vi "Identify Duplicate Alias Entries.vi"(8 "error in (no error)":errorcluster, 10 "Modified Index":i32, 11 "NewVal":T1[](array[typedef])) -> (0 "error out":errorcluster, 1 "Duplicate Message":string, 2 "Duplicate Entry":bool)   [LabVIEW 2020, in "Routing and Faulting System Explorer.lvlib"]
uses:
  Routing and Faulting System Explorer.lvlib
  Alias.ctl
  Endpoint.ctl
  Shared/Constants.vi
  Shared/Routing and Faulting Shared.lvlib
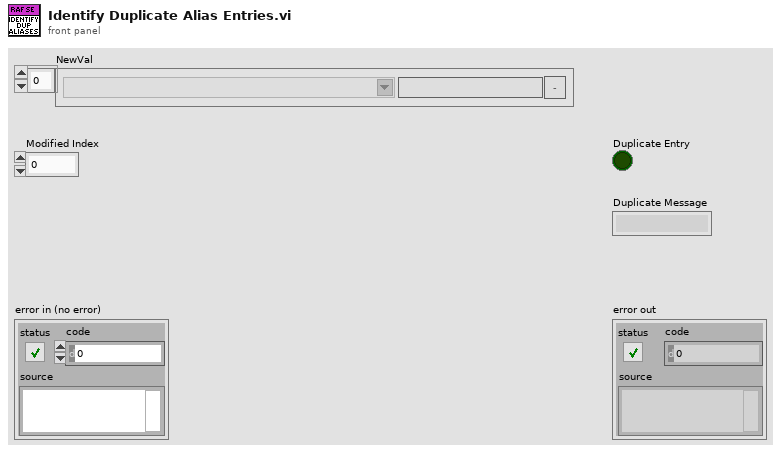
[diagram p1: front panel]
types:
  T1 = typedef "Routing and Faulting System Explorer.lvlib/Alias.ctl" = cluster{"Endpoint":T2, "Alias":string, "Remove":bool}
  T2 = typedef "Routing and Faulting System Explorer.lvlib/Endpoint.ctl" = string
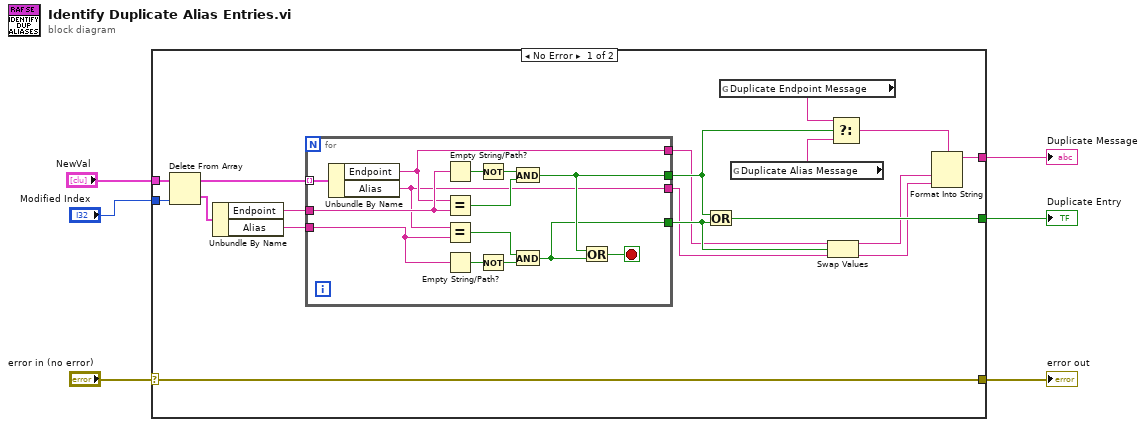
[diagram p0: block diagram]
diagram:
  n1 = case shown="No Error" "error in (no error)" {
    selector: "error in (no error)" -> [w7 w39]
    tunnel: "Modified Index" -> [w24 _]
    tunnel: "NewVal" -> [w23 _]
    tunnel: [w19 _] -> w4
    tunnel: [w10 _] -> w3
    tunnel: [w7 w39] -> w1
    frame No Error {
      n2 = Delete From Array(array=w23, index=w24) -> (deleted portion=w21:T1, array with subset deleted=w22:T1[])  [unwired: 1 in]
      n3 = Unbundle By Name(w21) -> ("Endpoint"=w15:T2, "Alias"=w14:string)
      n4 = for {
        tunnel: w22 -> [w38] mode=indexing
        tunnel: w15 -> [w27]
        tunnel: w14 -> [w28]
        tunnel: [w30] -> w20
        tunnel: [w29] -> w13
        tunnel: [w26] -> w8
        tunnel: [w25] -> w9
        stop <- w37 stop-if-true
        n5 = Unbundle By Name(w38) -> ("Endpoint"=w26:T2, "Alias"=w25:string)
        n6 = Empty String/Path?(string/path=w27) -> (empty?=w36:bool)
        n7 = Equal?(x=w26, y=w27) -> (x = y?=w34:bool)
        n8 = Equal?(x=w25, y=w28) -> (x = y?=w31:bool)
        n9 = Empty String/Path?(string/path=w28) -> (empty?=w33:bool)
        n10 = Not(x=w36) -> (.not. x?=w35:bool)
        n11 = Not(x=w33) -> (.not. x?=w32:bool)
        n12 = And(x=w35, y=w34) -> (x .and. y?=w30:bool)
        n13 = And(x=w31, y=w32) -> (x .and. y?=w29:bool)
        n14 = Or(x=w30, y=w29) -> (x .or. y?=w37:bool)
      }
      n15 = Or(x=w20, y=w13) -> (x .or. y?=w19:bool)
      n16 = global read "Constants.vi" "Duplicate Endpoint Message"() -> (w18:string)
      n17 = global read "Constants.vi" "Duplicate Alias Message"() -> (w17:string)
      n18 = Swap Values(12:w8, 13:w13, 14:w9) -> (1:w12:T2, 3:w11:string)
      n19 = Select(t=w18, s=w20, f=w17) -> (s? t:f=w16:string)
      n20 = Format Into String(format string=w16, w12, w11) -> (resulting string=w10:string)  [unwired: 2 in, 1 out]
    }
    frame Error {
    }
  }
  "error out" <- w1
  "Duplicate Entry" <- w4
  "Duplicate Message" <- w3
